vi "IDS Set Get Parameter.vi"(0 "IDS Notifier":refnum<notifier>, 5 "IDS Actions":T1, 7 "IDS Camera Ref":refnum<k24>, 11 "Error":errorcluster) -> (4 "IDS Notifier":refnum<notifier>, 15 "Error":errorcluster)   [LabVIEW 2025]
uses:
  IDS Controls/IDS Notifier Element.ctl
  IDS Controls/IDS Actions.ctl
  IDS Controls/IDS Parameters.ctl
  IDS Controls/IDS Parameter List.ctl
  IDS Controls/IDS ROI.ctl
  <vilib>/vision/Image Controls.llb/IMAQ Image.ctl
  C:/Users/Photonics03/Documents/Microscope-Control/Device Library/Cameras/IDS/IDS LabView Examples/LabVIEW/ueye.NET/uEyeDotNet.dll
  IDS LabView Examples/LabVIEW/ueye.NET/uEyeDotNet.dll
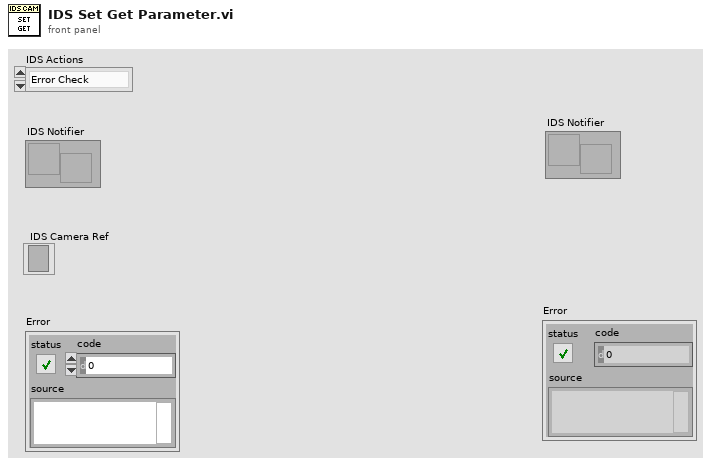
[diagram p1: front panel]
types:
  T1 = typedef "IDS Actions.ctl" = enum16{"Error Check", "Initialize", "Preview", "Record", "Abort", "Record Settings", "Set Parameter", "Get Parameter", "Set ROI", "Get ROI", "Status", "Quit"}
  T2 = typedef "IDS Notifier Element.ctl" = cluster{"IDS Actions":T1, "Received?":bool, "IDS Parameter":T3, "IDS ROI":T5, "Running?":bool, "File Path":path, "# of frames":u32, "Image Ref":T6, "Error":errorcluster, "Binning":i32}
  T3 = typedef "IDS Parameters.ctl" = cluster{"Parameter":T4, "Value":dbl}
  T4 = typedef "IDS Parameter List.ctl" = enum16{"Exposure Time (s)", "Binning"}
  T5 = typedef "IDS ROI.ctl" = cluster{"H Offset":i32, "V Offset":i32, "H Width":i32, "V Width":i32}
  T6 = typedef "IMAQ Image.ctl" = refnum<image>
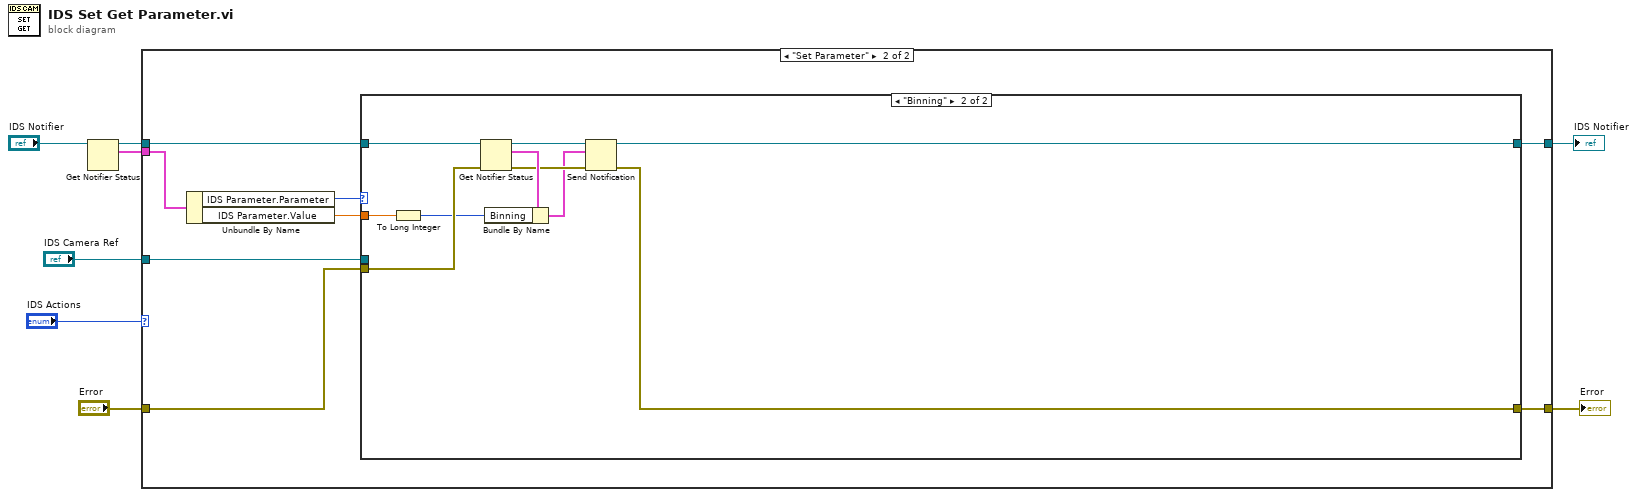
[diagram p0: block diagram]
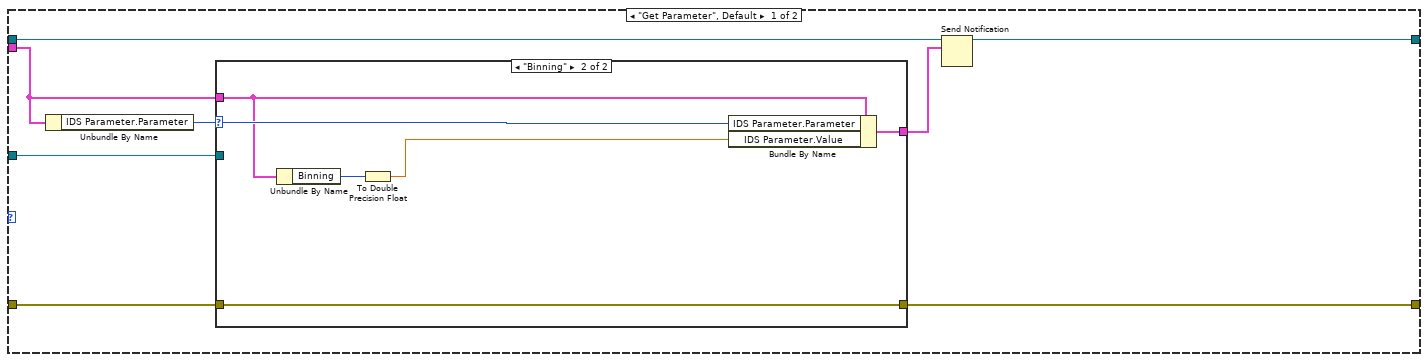
[diagram p2: hidden frame]
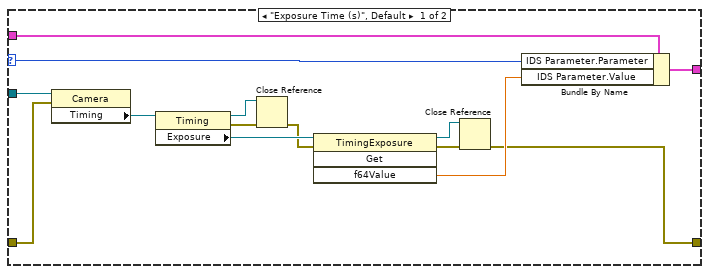
[diagram p3: hidden frame]
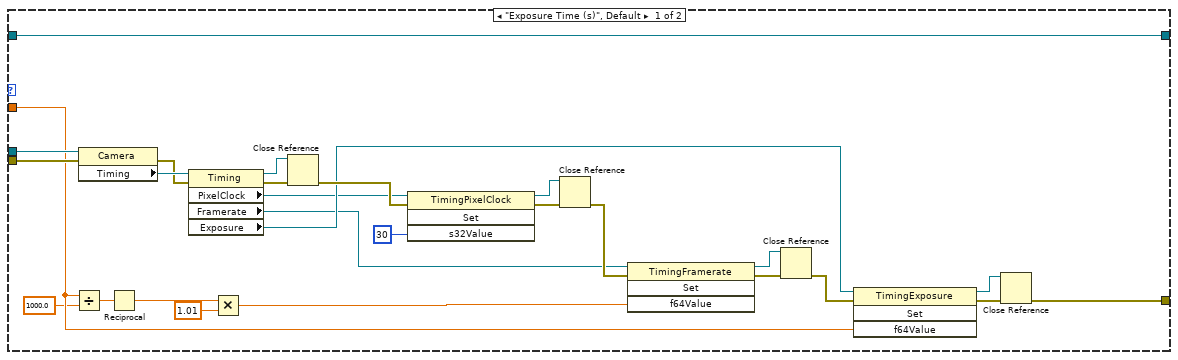
[diagram p4: hidden frame]
diagram:
  n1 = Get Notifier Status(notifier="IDS Notifier") -> (notifier out=w6:refnum<notifier>, current notification=w5:T2)  [unwired: 1 in, 3 out]
  n2 = case shown="\"Set Parameter\"" "IDS Actions" {
    tunnel: w6 -> [w11 w38]
    tunnel: w5 -> [w12 w44]
    tunnel: [w10 w37] -> w3
    tunnel: "IDS Camera Ref" -> [w13 w41]
    tunnel: "Error" -> [w15 w40]
    tunnel: [w14 w39] -> w1
    frame "Get Parameter", Default {
      n3 = Unbundle By Name(w12) -> ("IDS Parameter.Parameter"=w16:T4)
      n4 = case shown="\"Binning\"" w16 {
        selector: w16 -> [w21 w36]
        tunnel: w15 -> [w18 w33]
        tunnel: [w17 w33] -> w14
        tunnel: w13 -> [w30 _]
        tunnel: w12 -> [w22 w34]
        tunnel: [w19 w35] -> w9
        frame "Exposure Time (s)", Default {
          n5 = property class="Camera"(reference=w30, error in=w18) -> ("Timing"=w29:refnum<k24>)  [unwired: 2 out]
          n6 = property class="Timing"(reference=w29) -> (reference out=w27:refnum<k24>, error out=w26:errorcluster, "Exposure"=w28:refnum<k24>)  [unwired: 1 in]
          n7 = Close Reference(reference=w27, error in (no error)=w26) -> (error out=w25:errorcluster)
          n8 = invoke class="TimingExposure" method="Get"(reference=w28, error in=w25) -> (reference out=w24:refnum<k24>, error out=w23:errorcluster, "f64Value"=w20:dbl)  [unwired: 2 in, 1 out]
          n9 = Close Reference(reference=w24, error in (no error)=w23) -> (error out=w17:errorcluster)
          n10 = Bundle By Name(cluster=w22, "IDS Parameter.Parameter"=w21, "IDS Parameter.Value"=w20) -> (w19:T2)
        }
        frame "Binning" {
          n11 = Unbundle By Name(w34) -> ("Binning"=w32:i32)
          n12 = To Double Precision Float(number=w32) -> (double precision float=w31:dbl)
          n13 = Bundle By Name(cluster=w34, "IDS Parameter.Parameter"=w36, "IDS Parameter.Value"=w31) -> (w35:T2)
        }
      }
      n14 = Send Notification(notification=w9, notifier=w11) -> (notifier out=w10:refnum<notifier>)  [unwired: 1 in, 1 out]
    }
    frame "Set Parameter" {
      n15 = Unbundle By Name(w44) -> ("IDS Parameter.Parameter"=w43:T4, "IDS Parameter.Value"=w42:dbl)
      n16 = case shown="\"Binning\"" w43 {
        tunnel: w42 -> [w49 w81]
        tunnel: w41 -> [w55 _]
        tunnel: w40 -> [w56 w77]
        tunnel: [w52 w72] -> w39
        tunnel: w38 -> [w45 w80]
        tunnel: [w45 w73] -> w37
        frame "Exposure Time (s)", Default {
          n17 = Divide(x=w49, y=1000.0) -> (x/y=w48:dbl)
          n18 = property class="Camera"(reference=w55, error in=w56) -> (error out=w58:errorcluster, "Timing"=w59:refnum<k24>)  [unwired: 1 out]
          n19 = Reciprocal(x=w48) -> (1/x=w51:dbl)
          n20 = property class="Timing"(reference=w59, error in=w58) -> (reference out=w63:refnum<k24>, error out=w64:errorcluster, "PixelClock"=w60:refnum<k24>, "Framerate"=w61:refnum<k24>, "Exposure"=w62:refnum<k24>)
          n21 = Multiply(x=w51, y=1.01) -> (x*y=w46:dbl)
          n22 = Close Reference(reference=w63, error in (no error)=w64) -> (error out=w65:errorcluster)
          n23 = invoke class="TimingPixelClock" method="Set"(reference=w60, error in=w65, "s32Value"=30 ("Pixelclock")) -> (reference out=w68:refnum<k24>, error out=w66:errorcluster)  [unwired: 1 in, 2 out]
          n24 = Close Reference(reference=w68, error in (no error)=w66) -> (error out=w67:errorcluster)
          n25 = invoke on="Methodenknoten" class="TimingFramerate" method="Set"(reference=w61, error in=w67, "f64Value"=w46) -> (reference out=w71:refnum<k24>, error out=w69:errorcluster)  [unwired: 1 in, 2 out]
          n26 = Close Reference(reference=w71, error in (no error)=w69) -> (error out=w70:errorcluster)
          n27 = invoke class="TimingExposure" method="Set"(reference=w62, error in=w70, "f64Value"=w49) -> (reference out=w53:refnum<k24>, error out=w54:errorcluster)  [unwired: 1 in, 2 out]
          n28 = Close Reference(reference=w53, error in (no error)=w54) -> (error out=w52:errorcluster)
        }
        frame "Binning" {
          n29 = To Long Integer(number=w81) -> (32bit integer=w75:i32)
          n30 = Get Notifier Status(notifier=w80, error in (no error)=w77) -> (notifier out=w78:refnum<notifier>, current notification=w79:T2, error out=w76:errorcluster)  [unwired: 2 out]
          n31 = Bundle By Name(cluster=w79, "Binning"=w75) -> (w74:T2)
          n32 = Send Notification(notification=w74, notifier=w78, error in (no error)=w76) -> (notifier out=w73:refnum<notifier>, error out=w72:errorcluster)
        }
      }
    }
  }
  "IDS Notifier" <- w3
  "Error" <- w1
